vi "to variant.vi"(10 "Message":string, 11 "Variant":variant) -> (3 "Message Cluster":T1)   [LabVIEW 2015]
uses:
  PC/QMH Fundamentals - Message Cluster.ctl
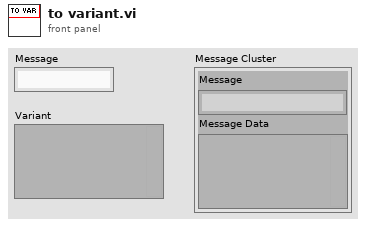
[diagram p1: front panel]
types:
  T1 = typedef "QMH Fundamentals - Message Cluster.ctl" = cluster{"Message":string, "Message Data":variant}
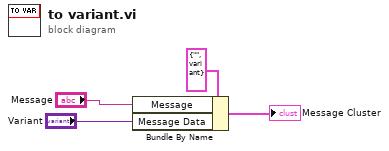
[diagram p0: block diagram]
diagram:
  n1 = Bundle By Name(cluster=T1 {"Message"="", "Message Data"=variant} ("Message Cluster"), "Message"="Message", "Message Data"="Variant") -> (→"Message Cluster":T1)
